vi "GUI.AutoSize.vi"(8 "error in (no error)":errorcluster, 11 "pathToMainVI in":path) -> (0 "error out":errorcluster, 3 "pathToMainVI out":path)   [LabVIEW 2019]
uses:
  <vilib>/Utility/miscctls.llb/LVPointTypeDef.ctl
  <vilib>/Utility/miscctls.llb/LVRectTypeDef.ctl
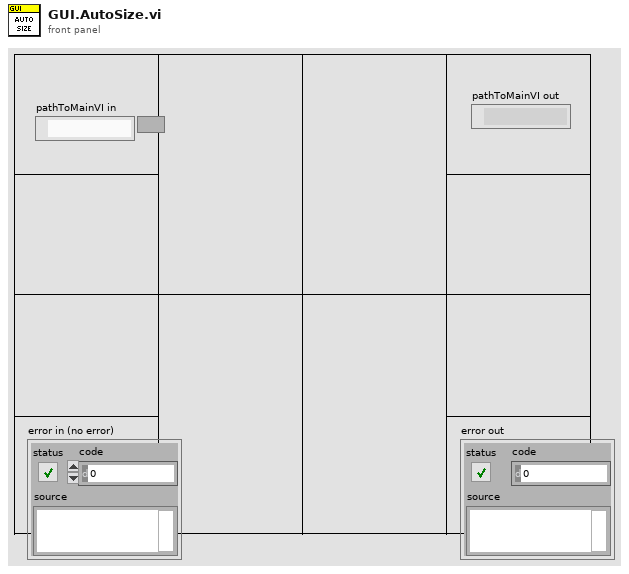
[diagram p1: front panel]
types:
  T1 = enum16{"Initialization", "Find Max Height", "Set Orgin", "Set Panel Bounds", "Center FP", "Shutdown"}
  T2 = typedef "LVPointTypeDef.ctl" = cluster{"Horizontal":i16, "Vertical":i16}
  T3 = typedef "LVRectTypeDef.ctl" = cluster{"Left":i16, "Top":i16, "Right":i16, "Bottom":i16}
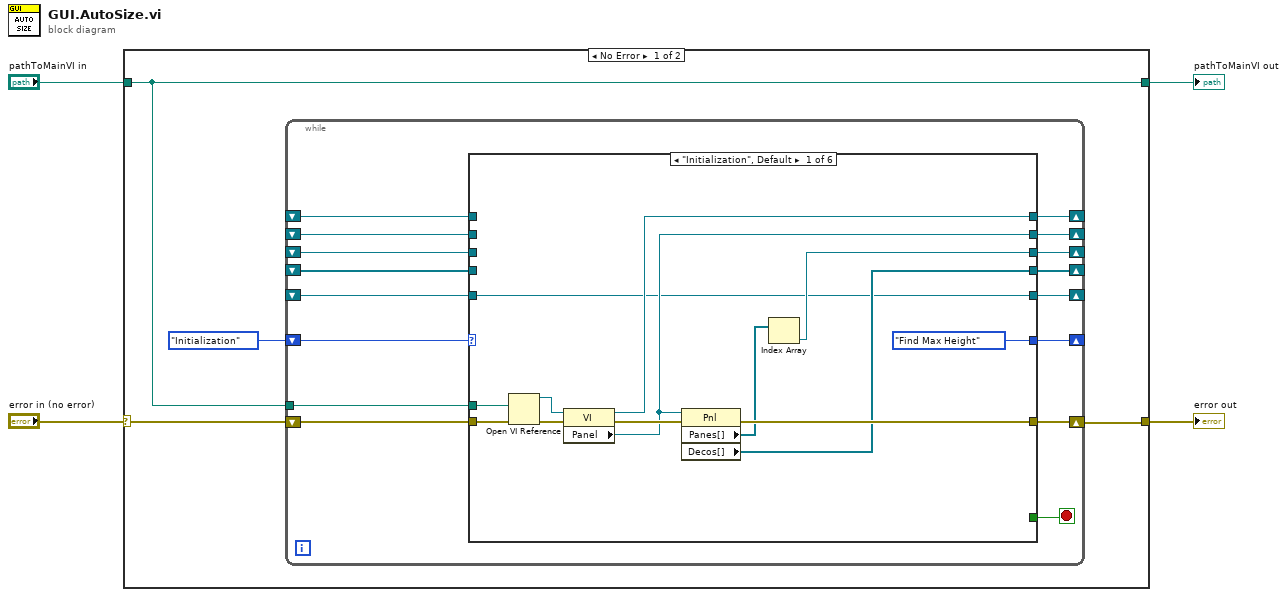
[diagram p0: block diagram]
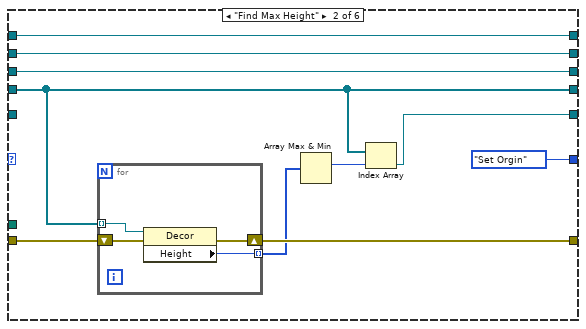
[diagram p2: hidden frame]
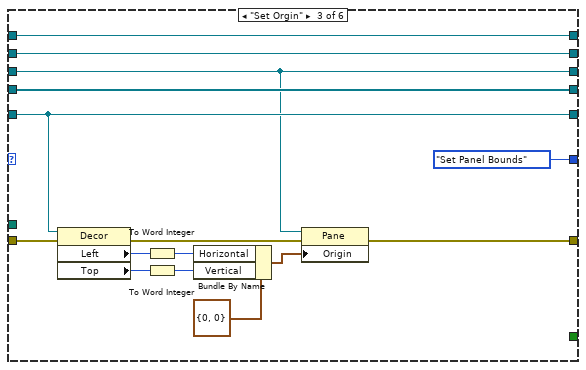
[diagram p3: hidden frame]
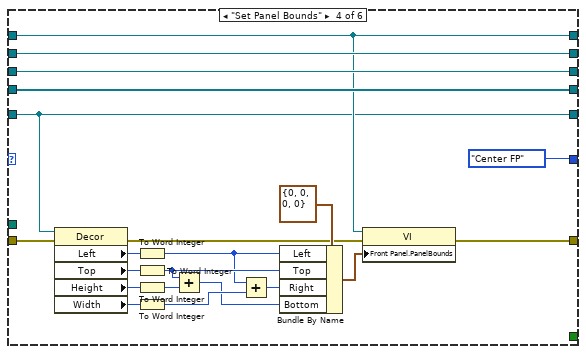
[diagram p4: hidden frame]
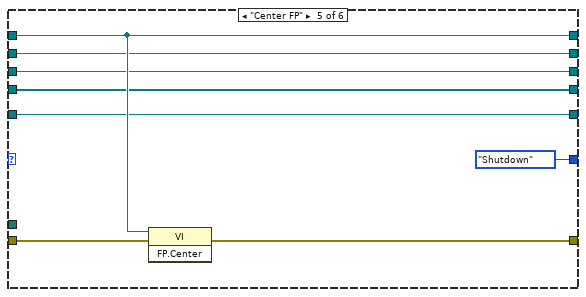
[diagram p5: hidden frame]
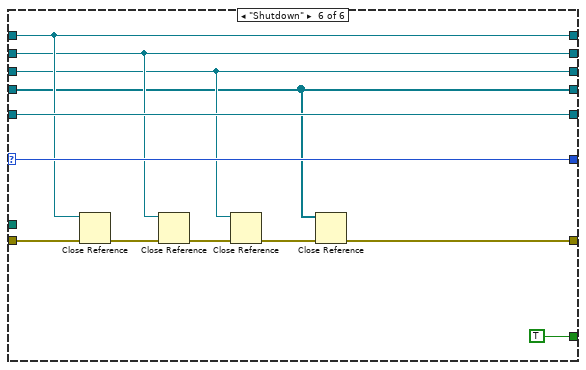
[diagram p6: hidden frame]
diagram:
  n1 = case shown="No Error" "error in (no error)" {
    selector: "error in (no error)" -> [w8 w108]
    tunnel: "pathToMainVI in" -> [w6 w109]
    tunnel: [w6 w109] -> w3
    tunnel: [w5 w108] -> w4
    frame No Error {
      n2 = while {
        shift-right: [w10] -> _
        shift-left: T1."Initialization" -> [w24]
        shift-right: [w23] -> w5
        shift-left: w8 -> [w22]
        tunnel: w6 -> [w21]
        shift-right: [w20] -> _
        shift-left: _ -> [w19]
        shift-right: [w18] -> _
        shift-left: _ -> [w17]
        shift-right: [w16] -> _
        shift-left: _ -> [w15]
        shift-right: [w14] -> _
        shift-left: _ -> [w13]
        shift-right: [w12] -> _
        shift-left: _ -> [w11]
        stop <- w9 stop-if-true
        n3 = case shown="\"Initialization\", Default" w24 {
          selector: w24 -> [_ _ _ _ _ w106]
          tunnel: [w30 w43 w53 w82 w94 w100] -> w23
          tunnel: w22 -> [w37 w44 w66 w84 w95 w105]
          tunnel: w21 -> [w36 _ _ _ _ _]
          tunnel: [w33 w47 w65 w83 w93 w104] -> w20
          tunnel: w19 -> [_ w47 w65 w83 w93 w104]
          tunnel: [w31 w46 w64 w87 w92 w99] -> w18
          tunnel: w17 -> [_ w46 w64 w87 w92 w99]
          tunnel: [w28 w45 w61 w86 w91 w98] -> w16
          tunnel: w15 -> [_ w45 w61 w86 w91 w98]
          tunnel: [w27 w41 w63 w85 w90 w97] -> w14
          tunnel: w13 -> [_ w41 w63 w85 w90 w97]
          tunnel: [w26 w39 w62 w76 w89 w107] -> w12
          tunnel: w11 -> [w26 _ w62 w76 w89 w107]
          tunnel: [T1."Find Max Height" T1."Set Orgin" T1."Set Panel Bounds" T1."Center FP" T1."Shutdown" w106] -> w10
          tunnel: [_ _ _ _ _ TRUE] -> w9
          frame "Initialization", Default {
            n4 = Open VI Reference(vi path=w36, error in (no error)=w37) -> (vi reference=w35:refnum<vi>, error out=w34:errorcluster)  [unwired: 4 in]
            n5 = property class="VI"(reference=w35, error in=w34) -> (reference out=w33:refnum<vi>, error out=w32:errorcluster, "Panel"=w31:refnum<vi>)
            n6 = property class="Pnl"(reference=w31, error in=w32) -> (error out=w30:errorcluster, "Panes[]"=w29:refnum<vi>[], "Decos[]"=w27:refnum<vi>[])  [unwired: 1 out]
            n7 = Index Array(array=w29) -> (element=w28:refnum<vi>)  [unwired: 1 in]
          }
          frame "Find Max Height" {
            n8 = for {
              shift-right: [w50] -> w43
              shift-left: w44 -> [w51]
              tunnel: w41 -> [w49] mode=indexing
              tunnel: [w48] -> w42 mode=indexing
              n9 = property class="Decor"(reference=w49, error in=w51) -> (error out=w50:errorcluster, "Height"=w48:u32)  [unwired: 1 out]
            }
            n10 = Array Max & Min(array=w42) -> (max index (indices)=w40:i32)  [unwired: 3 out]
            n11 = Index Array(array=w41, index=w40) -> (element=w39:refnum<vi>)
          }
          frame "Set Orgin" {
            n12 = property class="Decor"(reference=w62, error in=w66) -> (error out=w60:errorcluster, "Left"=w57:i32, "Top"=w58:i32)  [unwired: 1 out]
            n13 = To Word Integer(number=w57) -> (16bit integer=w56:i16)
            n14 = To Word Integer(number=w58) -> (16bit integer=w55:i16)
            n15 = Bundle By Name(cluster=T2 {"Horizontal"=0, "Vertical"=0} ("Origin"), "Horizontal"=w56, "Vertical"=w55) -> (w54:T2)
            n16 = property class="Pane"(reference=w61, error in=w60, "Origin"=w54) -> (error out=w53:errorcluster)  [unwired: 1 out]
          }
          frame "Set Panel Bounds" {
            n17 = property class="Decor"(reference=w76, error in=w84) -> (error out=w80:errorcluster, "Left"=w77:i32, "Top"=w78:i32, "Height"=w75:u32, "Width"=w74:u32)  [unwired: 1 out]
            n18 = To Word Integer(number=w77) -> (16bit integer=w71:i16)
            n19 = To Word Integer(number=w78) -> (16bit integer=w73:i16)
            n20 = To Word Integer(number=w75) -> (16bit integer=w72:i16)
            n21 = To Word Integer(number=w74) -> (16bit integer=w70:i16)
            n22 = Add(x=w73, y=w72) -> (x+y=w68:i16)
            n23 = Add(x=w71, y=w70) -> (x+y=w67:i16)
            n24 = Bundle By Name(cluster=T3 {"Left"=0, "Top"=0, "Right"=0, "Bottom"=0} ("Front Panel Window:Panel Bounds"), "Left"=w71, "Top"=w73, "Right"=w67, "Bottom"=w68) -> (w79:T3)
            n25 = property class="VI"(reference=w83, error in=w80, "Front Panel.PanelBounds"=w79) -> (error out=w82:errorcluster)  [unwired: 1 out]
          }
          frame "Center FP" {
            n26 = invoke class="VI" method="FP.Center"(reference=w93, error in=w95) -> (error out=w94:errorcluster)  [unwired: 1 in, 2 out]
          }
          frame "Shutdown" {
            n27 = Close Reference(reference=w104, error in (no error)=w105) -> (error out=w103:errorcluster)
            n28 = Close Reference(reference=w99, error in (no error)=w103) -> (error out=w102:errorcluster)
            n29 = Close Reference(reference=w98, error in (no error)=w102) -> (error out=w101:errorcluster)
            n30 = Close Reference(reference=w97, error in (no error)=w101) -> (error out=w100:errorcluster)
          }
        }
      }
    }
    frame Error {
    }
  }
  "error out" <- w4
  "pathToMainVI out" <- w3
